vi "S2DS_DetermineTargetInY.vi"(2 "Measurement ON?":bool, 3 "Scan parameters  in":T1 {"Y data taking" items=["in both direction", "in up direction only", "in down direction only"]; "X data taking" items=["in both direction", "in up direction only", "in down direction only"]}) -> (0 "Change y direction":bool, 1 "Scan parameters  out":T1 {"Y data taking" items=["in both direction", "in up direction only", "in down direction only"]; "X data taking" items=["in both direction", "in up direction only", "in down direction only"]})   [LabVIEW 2025]
uses:
  TYPE DEFS/S2DS_Sweep Info.ctl
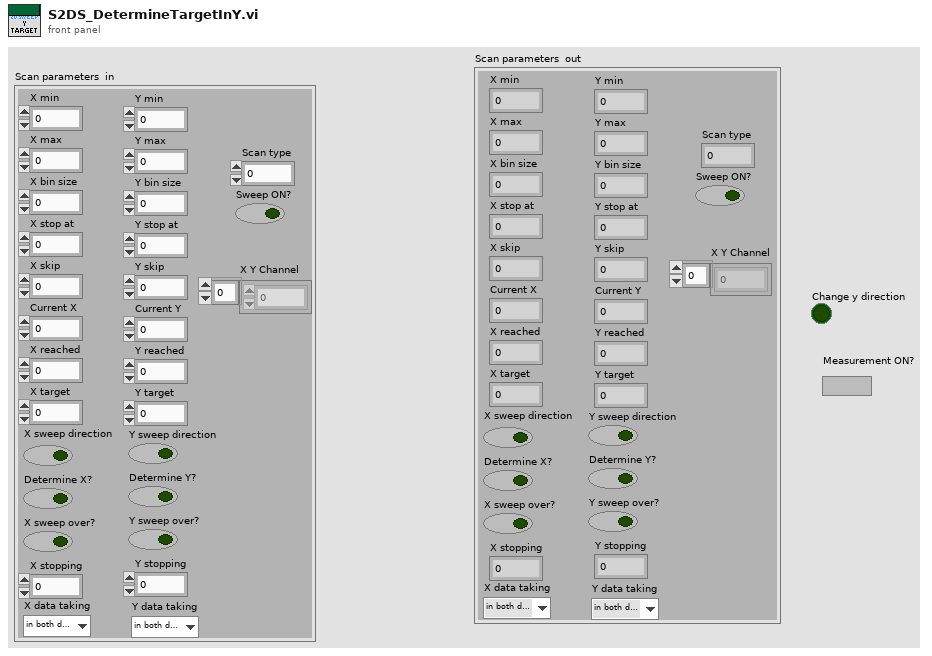
[diagram p1: front panel]
types:
  T1 = typedef "S2DS_Sweep Info.ctl" = cluster{"X min":ext, "X max":dbl, "Y min":dbl, "Y max":dbl, "X bin size":dbl, "Y bin size":dbl, "X stop at":dbl, "Y stop at":dbl, "X skip":u64, "Y skip":u64, "Current X":dbl, "Current Y":dbl, "X reached":i32, "Y reached":i32, "X target":dbl, "Y target":dbl, "Sweep ON?":bool, "X sweep direction":bool, "Y sweep direction":bool, "Determine X?":bool, "Determine Y?":bool, "X sweep over?":bool, "Y sweep over?":bool, "Scan type":i32, "X stopping":i32, "Y stopping":i32, "X Y Channel":u16[], "X data taking":u16, "Y data taking":u16}
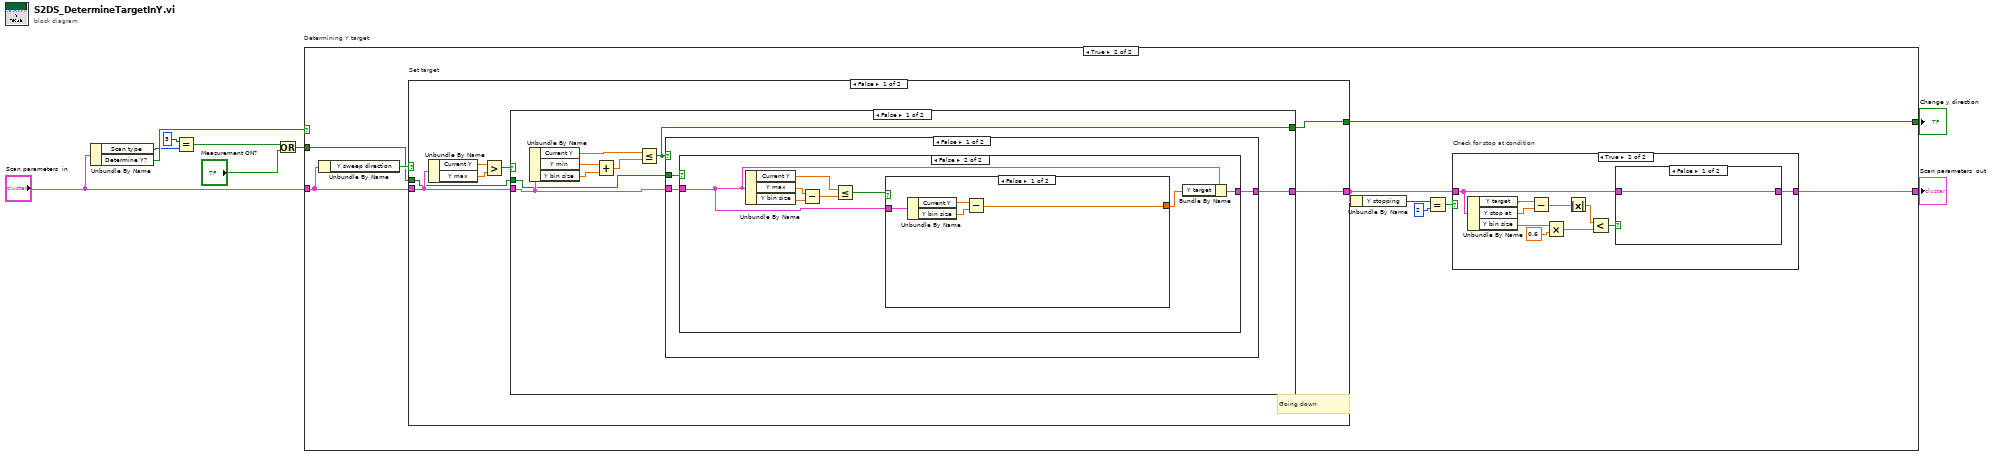
[diagram p0: block diagram]
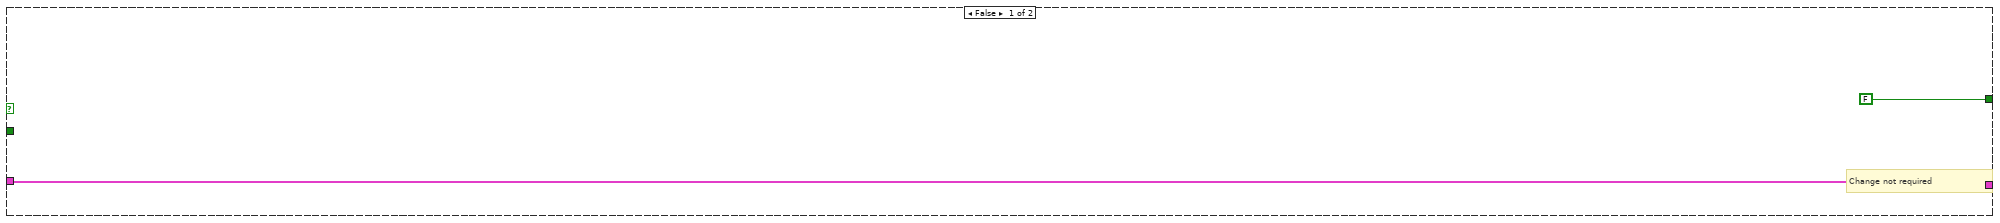
[diagram p2: hidden frame]
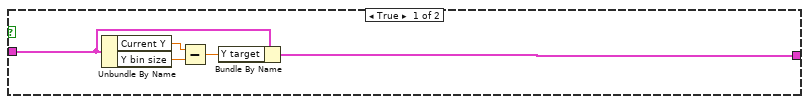
[diagram p3: hidden frame]
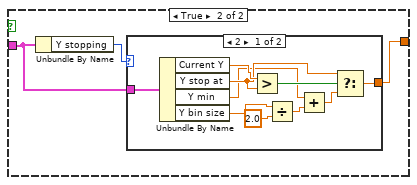
[diagram p4: hidden frame]
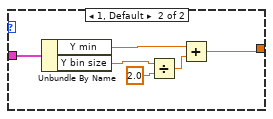
[diagram p5: hidden frame]
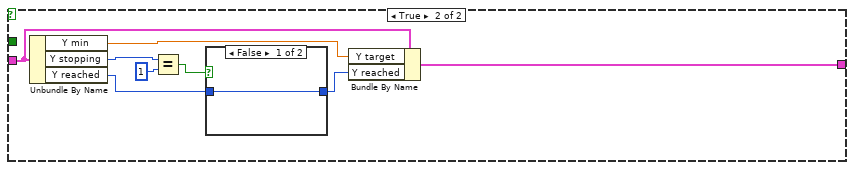
[diagram p6: hidden frame]
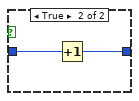
[diagram p7: hidden frame]
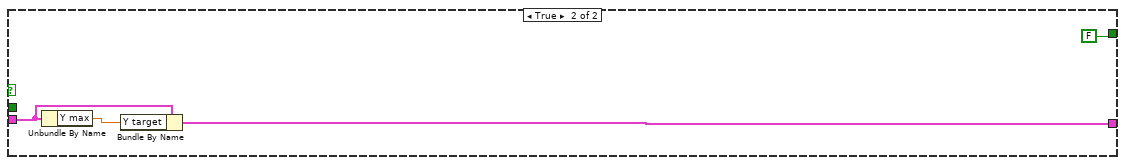
[diagram p8: hidden frame]
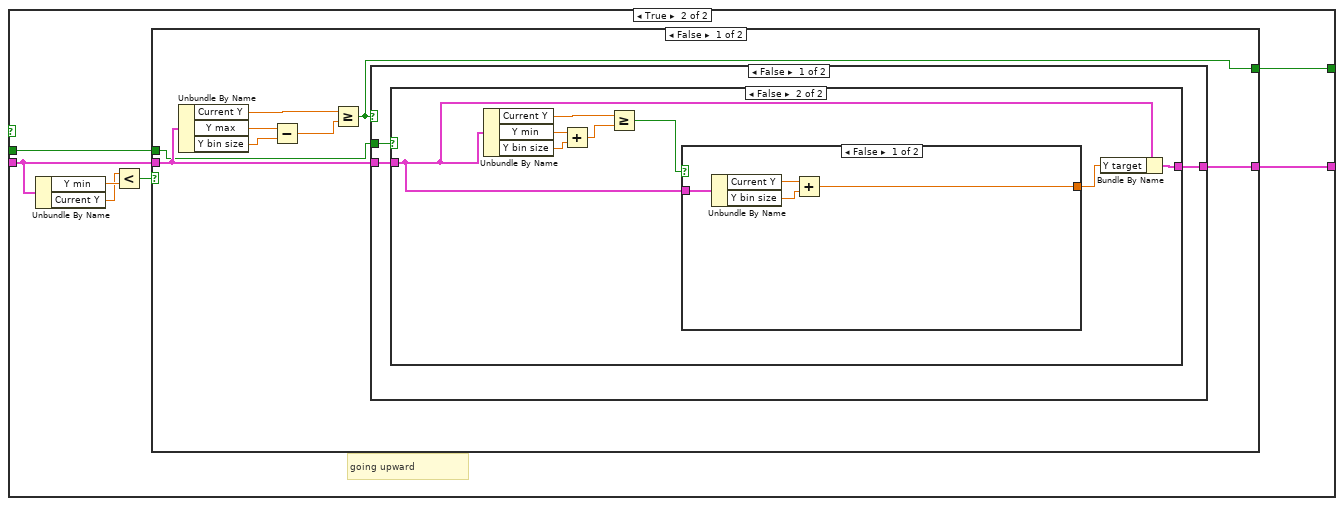
[diagram p9: hidden frame]
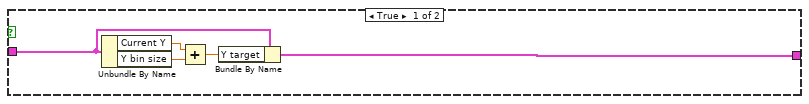
[diagram p10: hidden frame]
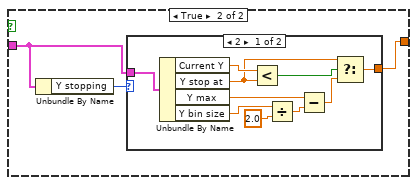
[diagram p11: hidden frame]
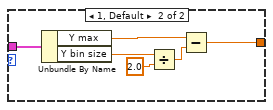
[diagram p12: hidden frame]
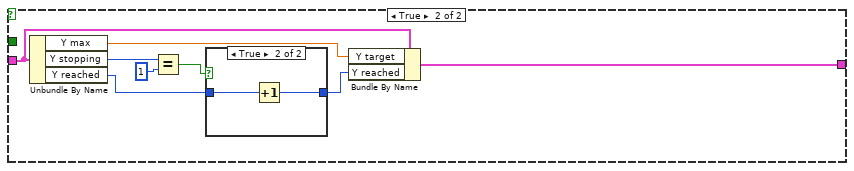
[diagram p13: hidden frame]
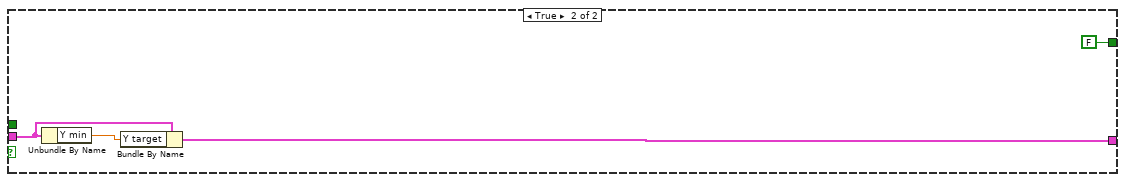
[diagram p15: hidden frame]
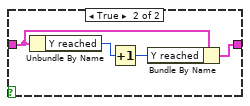
[diagram p17: hidden frame]
diagram:
  n1 = Unbundle By Name("Scan parameters  in") -> ("Scan type"=w5:i32, "Determine Y?"=w9:bool)
  n2 = Equal?(x=3, y=w5) -> (x = y?=w3:bool)
  n3 = Or(x=w3, y="Measurement ON?") -> (x .or. y?=w1:bool)
  n4 = case "Determining Y target" shown="True" w9 {
    tunnel: "Scan parameters  in" -> [w11 w20]
    tunnel: [w11 w14] -> w7
    tunnel: [FALSE w13] -> w6
    tunnel: w1 -> [_ w12]
    frame False {
      # "Change not required"
    }
    frame True {
      n5 = Unbundle By Name(w20) -> ("Y sweep direction"=w18:bool)
      n6 = case "Set target" shown="False" w18 {
        tunnel: w20 -> [w27 w93]
        tunnel: [w26 w92] -> w19
        tunnel: [w22 w91] -> w13
        tunnel: w12 -> [w21 w90]
        frame False {
          # "Going down"
          n7 = Unbundle By Name(w27) -> ("Current Y"=w25:dbl, "Y max"=w24:dbl)
          n8 = Greater?(x=w25, y=w24) -> (0:w23:bool)
          n9 = case shown="False" w23 {
            tunnel: w27 -> [w31 w89]
            tunnel: [w30 w87] -> w26
            tunnel: [w29 FALSE] -> w22
            tunnel: w21 -> [w28 _]
            frame False {
              n10 = Unbundle By Name(w31) -> ("Current Y"=w33:dbl, "Y min"=w35:dbl, "Y bin size"=w34:dbl)
              n11 = Add(x=w35, y=w34) -> (x+y=w32:dbl)
              n12 = Less Or Equal?(x=w33, y=w32) -> (x <= y?=w29:bool)
              n13 = case shown="False" w29 {
                tunnel: w31 -> [w38 w82]
                tunnel: [w37 w80] -> w30
                tunnel: w28 -> [w36 _]
                frame False {
                  n14 = case shown="False" w36 {
                    tunnel: w38 -> [w43 w49]
                    tunnel: [w42 w51] -> w37
                    frame True {
                      n15 = Unbundle By Name(w43) -> ("Current Y"=w41:dbl, "Y bin size"=w40:dbl)
                      n16 = Subtract(x=w41, y=w40) -> (x-y=w39:dbl)
                      n17 = Bundle By Name(cluster=w43, "Y target"=w39) -> (w42:T1)
                    }
                    frame False {
                      n18 = Unbundle By Name(w49) -> ("Current Y"=w45:dbl, "Y max"=w48:dbl, "Y bin size"=w47:dbl)
                      n19 = Subtract(x=w48, y=w47) -> (x-y=w46:dbl)
                      n20 = Less Or Equal?(x=w45, y=w46) -> (x <= y?=w44:bool)
                      n21 = case shown="False" w44 {
                        tunnel: [w52 w58] -> w50
                        tunnel: w49 -> [w53 w57]
                        frame False {
                          n22 = Unbundle By Name(w53) -> ("Current Y"=w55:dbl, "Y bin size"=w54:dbl)
                          n23 = Subtract(x=w55, y=w54) -> (x-y=w52:dbl)
                        }
                        frame True {
                          n24 = Unbundle By Name(w57) -> ("Y stopping"=w56:i32)
                          n25 = case shown="2" w56 {
                            tunnel: w57 -> [w68 w74]
                            tunnel: [w59 w72] -> w58
                            frame 2 {
                              n26 = Unbundle By Name(w68) -> ("Current Y"=w67:dbl, "Y stop at"=w65:dbl, "Y min"=w64:dbl, "Y bin size"=w63:dbl)
                              n27 = Greater?(x=w67, y=w65) -> (0:w66:bool)
                              n28 = Divide(x=w63, y=2.0) -> (x/y=w62:dbl)
                              n29 = Add(x=w64, y=w62) -> (x+y=w60:dbl)
                              n30 = Select(t=w65, s=w66, f=w60) -> (s? t:f=w59:dbl)
                            }
                            frame 1, Default {
                              n31 = Unbundle By Name(w74) -> ("Y min"=w73:dbl, "Y bin size"=w71:dbl)
                              n32 = Divide(x=w71, y=2.0) -> (x/y=w69:dbl)
                              n33 = Add(x=w73, y=w69) -> (x+y=w72:dbl)
                            }
                          }
                        }
                      }
                      n34 = Bundle By Name(cluster=w49, "Y target"=w50) -> (w51:T1)
                    }
                  }
                }
                frame True {
                  n35 = Unbundle By Name(w82) -> ("Y min"=w81:dbl, "Y stopping"=w75:i32, "Y reached"=w79:i32)
                  n36 = Equal?(x=w75, y=1) -> (x = y?=w76:bool)
                  n37 = case shown="False" w76 {
                    tunnel: w79 -> [w83 w85]
                    tunnel: [w83 w84] -> w78
                    frame False {
                    }
                    frame True {
                      n38 = Increment(x=w85) -> (x+1=w84:i32)
                    }
                  }
                  n39 = Bundle By Name(cluster=w82, "Y target"=w81, "Y reached"=w78) -> (w80:T1)
                }
              }
            }
            frame True {
              n40 = Unbundle By Name(w89) -> ("Y max"=w88:dbl)
              n41 = Bundle By Name(cluster=w89, "Y target"=w88) -> (w87:T1)
            }
          }
        }
        frame True {
          # "going upward"
          n42 = Unbundle By Name(w93) -> ("Y min"=w96:dbl, "Current Y"=w95:dbl)
          n43 = Less?(x=w95, y=w96) -> (x < y?=w94:bool)
          n44 = case shown="False" w94 {
            tunnel: w93 -> [w100 w158]
            tunnel: [w99 w156] -> w92
            tunnel: [w98 FALSE] -> w91
            tunnel: w90 -> [w97 _]
            frame False {
              n45 = Unbundle By Name(w100) -> ("Current Y"=w102:dbl, "Y max"=w104:dbl, "Y bin size"=w103:dbl)
              n46 = Subtract(x=w104, y=w103) -> (x-y=w101:dbl)
              n47 = Greater Or Equal?(x=w102, y=w101) -> (x >= y?=w98:bool)
              n48 = case shown="False" w98 {
                tunnel: w100 -> [w107 w151]
                tunnel: [w106 w149] -> w99
                tunnel: w97 -> [w105 _]
                frame False {
                  n49 = case shown="False" w105 {
                    tunnel: w107 -> [w112 w114]
                    tunnel: [w111 w120] -> w106
                    frame True {
                      n50 = Unbundle By Name(w112) -> ("Current Y"=w110:dbl, "Y bin size"=w109:dbl)
                      n51 = Add(x=w110, y=w109) -> (x+y=w108:dbl)
                      n52 = Bundle By Name(cluster=w112, "Y target"=w108) -> (w111:T1)
                    }
                    frame False {
                      n53 = Unbundle By Name(w114) -> ("Current Y"=w115:dbl, "Y min"=w118:dbl, "Y bin size"=w117:dbl)
                      n54 = Add(x=w118, y=w117) -> (x+y=w116:dbl)
                      n55 = Greater Or Equal?(x=w115, y=w116) -> (x >= y?=w113:bool)
                      n56 = case shown="False" w113 {
                        tunnel: [w121 w127] -> w119
                        tunnel: w114 -> [w124 w126]
                        frame False {
                          n57 = Unbundle By Name(w124) -> ("Current Y"=w123:dbl, "Y bin size"=w122:dbl)
                          n58 = Add(x=w123, y=w122) -> (x+y=w121:dbl)
                        }
                        frame True {
                          n59 = Unbundle By Name(w126) -> ("Y stopping"=w125:i32)
                          n60 = case shown="2" w125 {
                            tunnel: w126 -> [w137 w143]
                            tunnel: [w128 w141] -> w127
                            frame 2 {
                              n61 = Unbundle By Name(w137) -> ("Current Y"=w136:dbl, "Y stop at"=w134:dbl, "Y max"=w133:dbl, "Y bin size"=w132:dbl)
                              n62 = Less?(x=w136, y=w134) -> (x < y?=w135:bool)
                              n63 = Divide(x=w132, y=2.0) -> (x/y=w130:dbl)
                              n64 = Subtract(x=w133, y=w130) -> (x-y=w129:dbl)
                              n65 = Select(t=w134, s=w135, f=w129) -> (s? t:f=w128:dbl)
                            }
                            frame 1, Default {
                              n66 = Unbundle By Name(w143) -> ("Y max"=w142:dbl, "Y bin size"=w140:dbl)
                              n67 = Divide(x=w140, y=2.0) -> (x/y=w138:dbl)
                              n68 = Subtract(x=w142, y=w138) -> (x-y=w141:dbl)
                            }
                          }
                        }
                      }
                      n69 = Bundle By Name(cluster=w114, "Y target"=w119) -> (w120:T1)
                    }
                  }
                }
                frame True {
                  n70 = Unbundle By Name(w151) -> ("Y max"=w150:dbl, "Y stopping"=w144:i32, "Y reached"=w148:i32)
                  n71 = Equal?(x=w144, y=1) -> (x = y?=w145:bool)
                  n72 = case shown="True" w145 {
                    tunnel: w148 -> [w152 w154]
                    tunnel: [w152 w153] -> w147
                    frame False {
                    }
                    frame True {
                      n73 = Increment(x=w154) -> (x+1=w153:i32)
                    }
                  }
                  n74 = Bundle By Name(cluster=w151, "Y target"=w150, "Y reached"=w147) -> (w149:T1)
                }
              }
            }
            frame True {
              n75 = Unbundle By Name(w158) -> ("Y min"=w157:dbl)
              n76 = Bundle By Name(cluster=w158, "Y target"=w157) -> (w156:T1)
            }
          }
        }
      }
      n77 = Unbundle By Name(w19) -> ("Y stopping"=w15:i32)
      n78 = Equal?(x=w15, y=2) -> (x = y?=w16:bool)
      n79 = case "Check for stop at condition" shown="True" w16 {
        tunnel: w19 -> [w159 w161]
        tunnel: [w159 w160] -> w14
        frame False {
        }
        frame True {
          n80 = Unbundle By Name(w161) -> ("Y target"=w169:dbl, "Y stop at"=w168:dbl, "Y bin size"=w165:dbl)
          n81 = Subtract(x=w169, y=w168) -> (x-y=w167:dbl)
          n82 = Multiply(x=w165, y=0.6) -> (x*y=w163:dbl)
          n83 = Absolute Value(x=w167) -> (abs(x)=w164:dbl)
          n84 = Less?(x=w164, y=w163) -> (x < y?=w162:bool)
          n85 = case shown="False" w162 {
            tunnel: w161 -> [w170 w173]
            tunnel: [w170 w172] -> w160
            frame False {
            }
            frame True {
              n86 = Unbundle By Name(w173) -> ("Y reached"=w174:i32)
              n87 = Increment(x=w174) -> (x+1=w171:i32)
              n88 = Bundle By Name(cluster=w173, "Y reached"=w171) -> (w172:T1)
            }
          }
        }
      }
    }
  }
  "Scan parameters  out" <- w7
  "Change y direction" <- w6
